vi "Turret Logic.vi"(8 "Vision Target?":bool, 9 "Vision Xoffset":dbl, 10 "Shooting Position":T2, 11 "Driver Xoffset":dbl) -> (0 "Activate vision":bool, 1 "Turret Offset(degrees)":dbl, 2 "Turret mode":T1=enum."IMU", 3 "Scan Mode":bool, 5 "Turret In Range?":bool)   [LabVIEW 2019, in "Robot.lvlib" / "Panzer.lvclass"]
uses:
  Panzer.lvclass
  Turret/Controls/Turret control states.ctl
  Turret/Turret.lvclass
  PowerCellHandler/Controls/Shooting Position.ctl
  PowerCellHandler/Power Cell Handler.lvclass
  <vilib>/Rock Robotics/Network Tables/NT Write String.vi
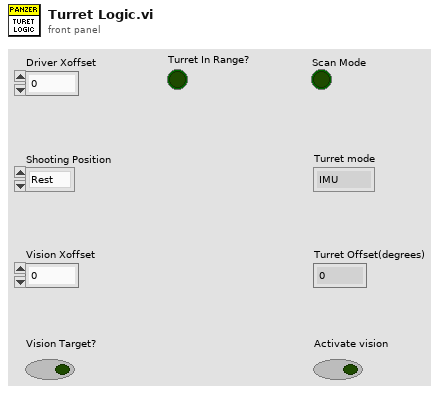
[diagram p1: front panel]
types:
  T1 = typedef "Turret.lvlib/Turret.lvclass/Turret control states.ctl" = enum16{"Position", "Offset", "IMU"}
  T2 = typedef "Power Cell Handler.lvlib/Power Cell Handler.lvclass/Shooting Position.ctl" = enum16{"Rest", "Front", "Middle", "Back"}
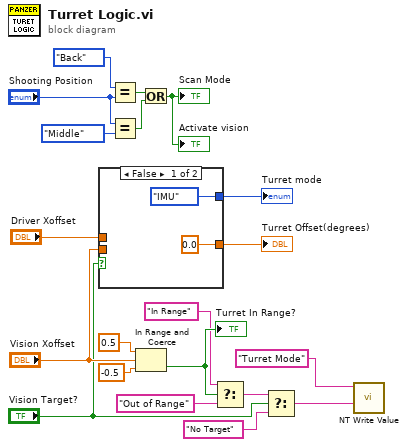
[diagram p0: block diagram]
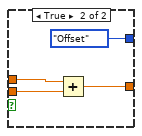
[diagram p2: hidden frame]
diagram:
  n1 = case shown="False" "Vision Target?" {
    tunnel: [0.0 ("f") w23] -> w15
    tunnel: "Vision Xoffset" -> [_ w24]
    tunnel: [Turret_control_states."IMU" ("Turret mode") Turret_control_states."Offset" ("Turret mode")] -> w14
    tunnel: "Driver Xoffset" -> [_ w25]
    frame False {
    }
    frame True {
      n2 = Add(x=w25, y=w24) -> (x+y=w23:dbl)
    }
  }
  "Turret Offset(degrees)" <- w15
  "Turret mode" <- w14
  n3 = Equal?(x=Shooting_Position."Back" ("Shooting Position"), y="Shooting Position") -> (x = y?=w17:bool)
  n4 = Equal?(x="Shooting Position", y=Shooting_Position."Middle" ("Shooting Position")) -> (x = y?=w16:bool)
  n5 = In Range and Coerce(upper limit=0.5, x="Vision Xoffset", lower limit=-0.5) -> (In Range?=w6:bool)  [unwired: 1 out]
  "Turret In Range?" <- w6
  n6 = Or(x=w17, y=w16) -> (x .or. y?=→"Activate vision" →"Scan Mode":bool)
  n7 = Select(t="In Range", s=w6, f="Out of Range") -> (s? t:f=w7:string)
  n8 = Select(t=w7, s="Vision Target?", f="No Target") -> (s? t:f=w2:string)
  n9 = call-poly <vilib>:"NT Write Value.vi"("String"=w2, "Name"="Turret Mode") -> ()  [unwired: 9 in, 1 out]
